vi "SCMP - flip array horizontally.vi"(11 "A in":u32[][](array[numeric])) -> (3 "A out":u32[][](array[numeric]))   [LabVIEW 2014]
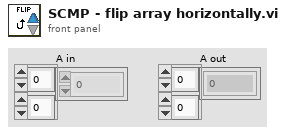
[diagram p1: front panel]
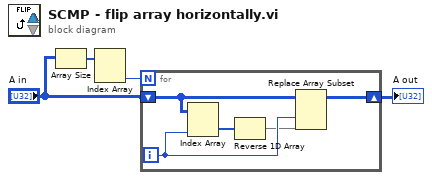
[diagram p0: block diagram]
diagram:
  n1 = Array Size(array="A in") -> (size(s)=w1:i32[])
  n2 = Index Array(array=w1) -> (element #2=w2:i32)  [unwired: 2 in, 1 out]
  n3 = for {
    N: w2 -> [_]
    shift-right: [w8] -> w4
    shift-left: "A in" -> [w7]
    i -> [w9]
    n4 = Index Array(array=w7, index (col)=w9) -> (element=w6:u32[])  [unwired: 1 in]
    n5 = Reverse 1D Array(array=w6) -> (reversed array=w5:u32[])
    n6 = Replace Array Subset(array=w7, new element=w5, index (col)=w9) -> (w8:u32[][])  [unwired: 1 in]
  }
  "A out" <- w4
